vi "Get UI Details.vi"(8 "error in":errorcluster, 11 "gRPC Server in":refnum<class "MeasurementPluginService.lvclass">) -> (0 "error out":errorcluster, 2 "user_interface_details":T1[](array[typedef]), 3 "gRPC Server out":refnum<class "MeasurementPluginService.lvclass">)   [LabVIEW 2020, in "MeasurementLink Measurement Server.lvlib" / "MeasurementPluginService.lvclass"]
uses:
  MeasurementPluginService.lvclass
  MeasurementLink Measurement Server Internal/RPC Messages/ni_measurementlink_measurement_v1_UserInterfaceDetails.ctl
  MeasurementLink Measurement Server Internal/MeasurementLink Measurement Server Internal.lvlib
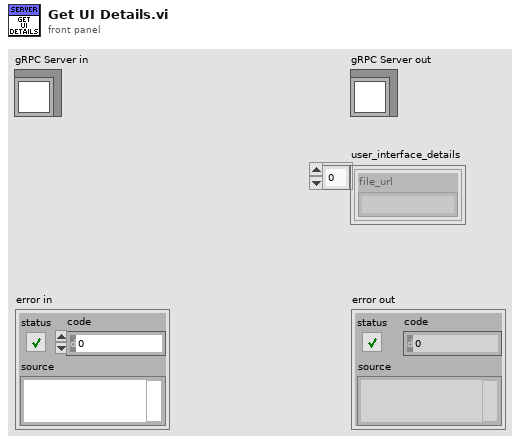
[diagram p1: front panel]
types:
  T1 = typedef "MeasurementLink Measurement Server Internal.lvlib/ni_measurementlink_measurement_v1_UserInterfaceDetails.ctl" = cluster{"file_url":string}
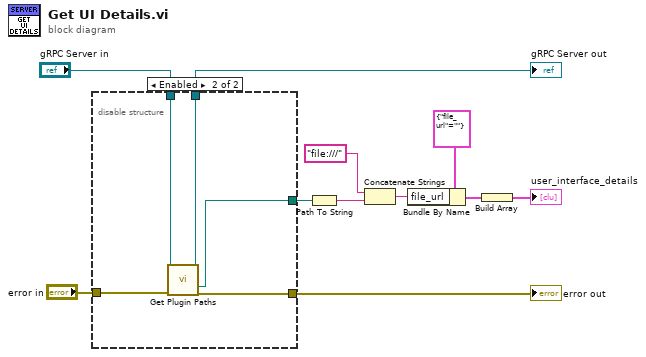
[diagram p0: block diagram]
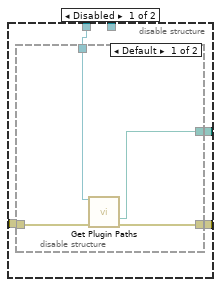
[diagram p2: hidden frame]
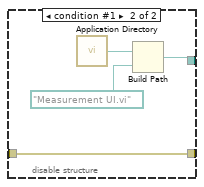
[diagram p3: hidden frame]
diagram:
  n1 = disable-structure shown="Enabled" {
    disable-tunnel: [w15 w25] -> w7
    disable-tunnel: "error in" -> [w14 w26]
    disable-tunnel: [w13 w28] -> w5
    disable-tunnel: "gRPC Server in" -> [w12 w27]
    disable-tunnel: [_ w24] -> w1
    frame Disabled {
      n2 = disable-structure shown="Default" {
        disable-tunnel: w14 -> [w19 w20]
        disable-tunnel: [w18 w20] -> w13
        disable-tunnel: [w16 w21] -> w15
        disable-tunnel: w12 -> [w17 _]
        frame condition #0 (active) {
          n3 = call-dynamic "Get Plugin Paths.vi"("MeasurementService in"=w17, "error in (no error)"=w19) -> ("Measurement UI VI Path"=w16:path, "error out"=w18:errorcluster)  [unwired: 7 in, 5 out]
        }
        frame condition #1 {
          n4 = call <vilib>:"Application Directory.vi"() -> ("Application Directory"=w23:path)
          n5 = Build Path(base path=w23, name or relative path=path "Measurement UI.vi") -> (appended path=w21:path)
        }
      }
    }
    frame Enabled {
      n6 = call-dynamic "Get Plugin Paths.vi"("MeasurementService in"=w27, "error in (no error)"=w26) -> ("MeasurementService out"=w24:refnum<class "MeasurementPluginService.lvclass">, "Measurement UI VI Path"=w25:path, "error out"=w28:errorcluster)  [unwired: 7 in, 4 out]
    }
  }
  "error out" <- w5
  "gRPC Server out" <- w1
  n7 = Path To String(path=w7) -> (string=w10:string)
  n8 = Concatenate Strings("file:///" ("string"), w10) -> (w9:string)
  n9 = Bundle By Name(cluster=T1 {"file_url"=""} ("UserInterfaceDetails"), "file_url"=w9) -> (w4:T1)
  n10 = Build Array(w4) -> (→"user_interface_details":T1[])
